vi "pf_Get_3D-Data_3D03.vi"(7 "Aquired Image":T1, 8 "error in (no error)":errorcluster, 9 "FrameCombine_NrOfFrames":u32, 10 "FrameCombine_Enable":bool=TRUE, 11 "PeakDetector_Mode":u32) -> (0 "error out":errorcluster, 1 "Quality Profile":u8[][](array[numeric]), 2 "Width Profile":u8[][](array[numeric]), 3 "Peak Profile":sgl[][](array[numeric]), 4 "Linescan":u8[][](array[numeric]), 5 "Status Line":u8[][](array[numeric]))   [LabVIEW 2012, in "Photonfocus_Toolkit.lvlib"]
uses:
  <userlib>/Photonfocus Toolkit/Photonfocus_Toolkit.lvlib
  <vilib>/vision/Image Controls.llb/IMAQ Image.ctl
  <vilib>/Analysis/Matrix/Numeric/Conversions/Array To Matrix - RA2.vi
  <vilib>/Analysis/Matrix/Numeric/Conversions/Matrix To Array - RM.vi
  <vilib>/Analysis/Matrix/NI_Matrix.lvlib
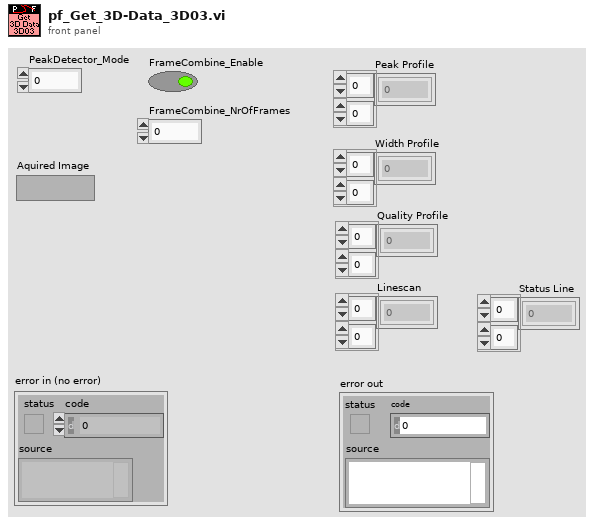
[diagram p1: front panel]
types:
  T1 = typedef "IMAQ Image.ctl" = refnum<image>
  T2 = enum8{"2D only", "2D and 3D", "3D only", "Undefined"}
  T3 = typedef "NI_Matrix.lvlib/RealMatrix.ctl" = dbl[][]
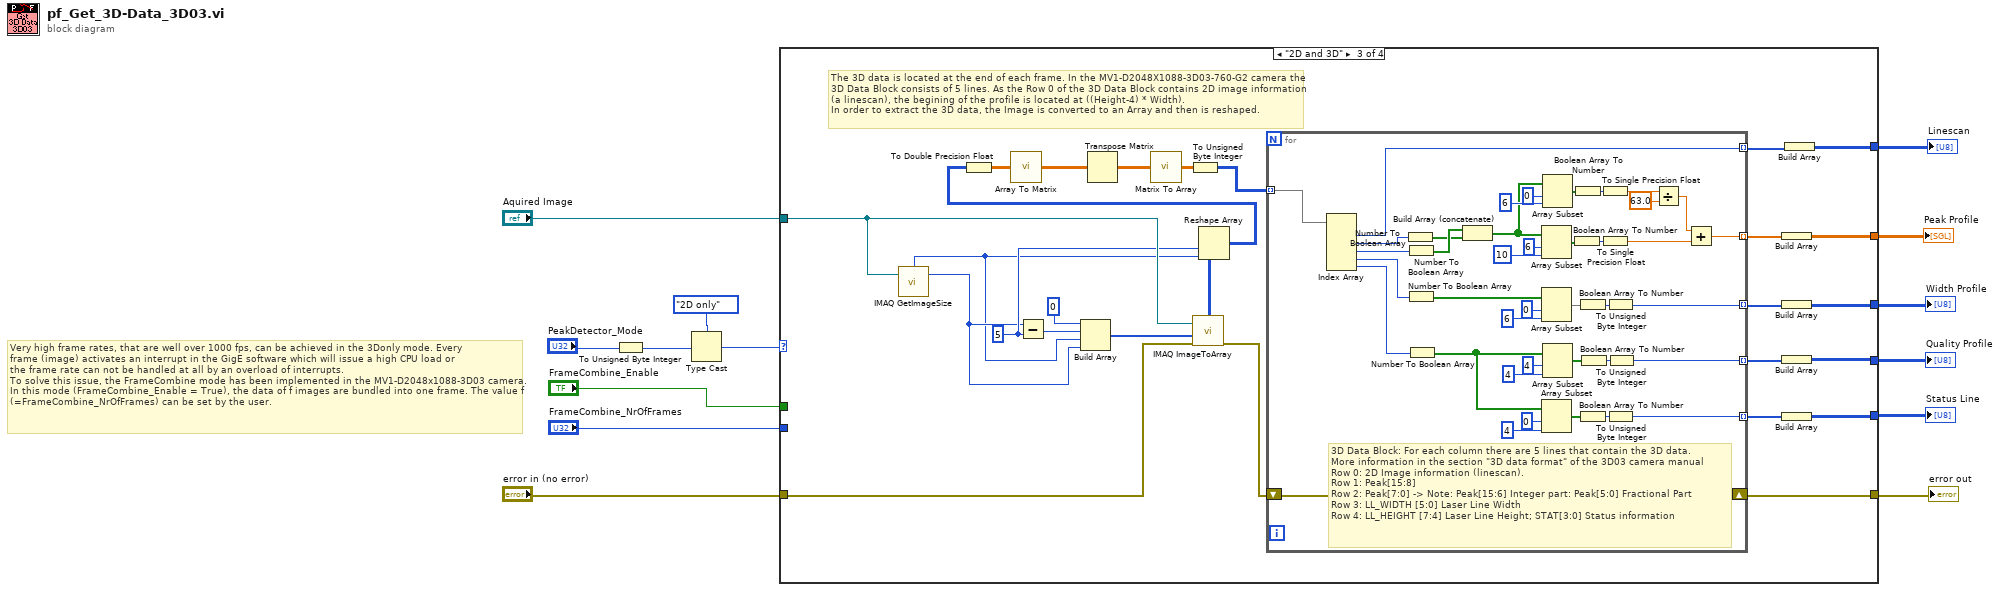
[diagram p0: block diagram]
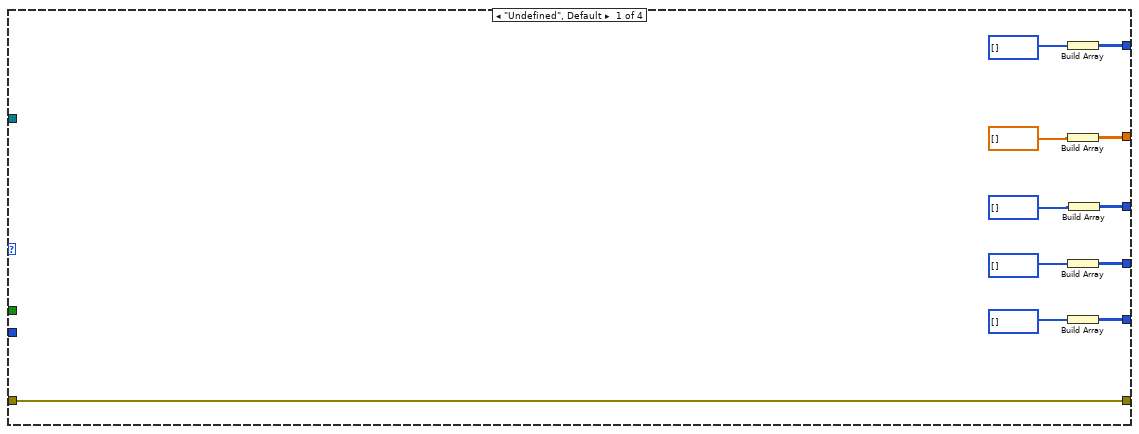
[diagram p2: hidden frame]
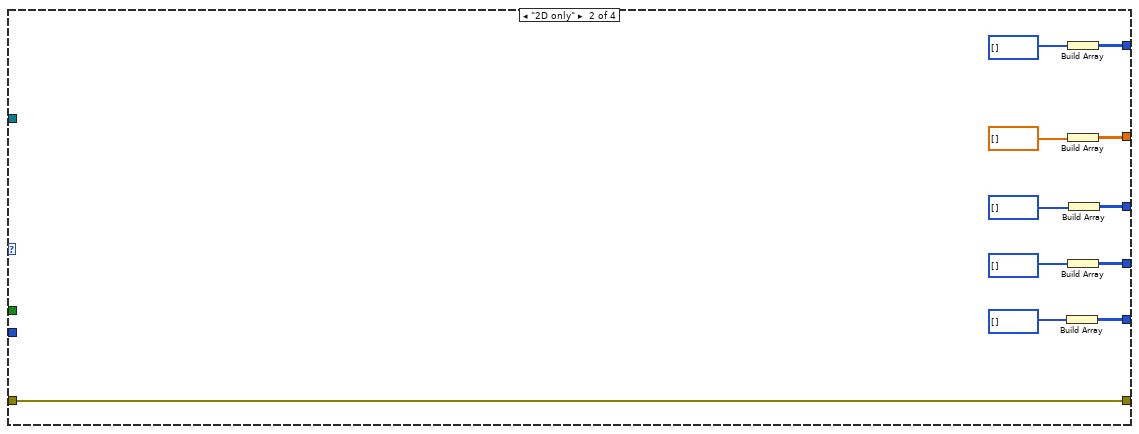
[diagram p3: hidden frame]
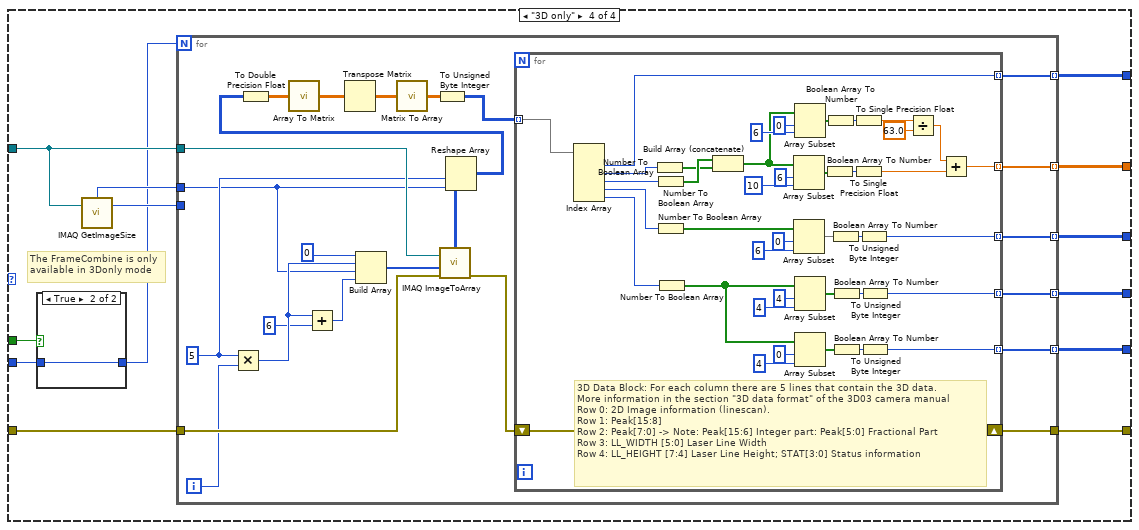
[diagram p4: hidden frame]
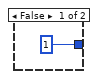
[diagram p5: hidden frame]
diagram:
  # "Very high frame rates, that are well over 1000 fps, can be achieved in the 3Donly mode. Every\nframe (image) activates an interrupt in the GigE software which will issue a high CPU load or\nthe frame rate can not be handled at all by an overload of interrupts.\nTo solve this issue, the FrameCombine mode has been implemented in the MV1-D2048x1088-3D03 camera. In this mode (FrameCombine_Enable = True), the data of f images are bundled into one frame. The value f (=FrameCombine_NrOfFrames) can be set by the user."
  n1 = To Unsigned Byte Integer(number="PeakDetector_Mode") -> (unsigned 8bit integer=w7:u8)
  n2 = Type Cast(type=T2."2D only", x=w7) -> (*(type *) &x=w9:T2)
  n3 = case shown="\"2D and 3D\"" w9 {
    tunnel: "Aquired Image" -> [_ _ w56 w116]
    tunnel: [w21 w34 w47 w112] -> w5
    tunnel: [w20 w32 w45 w111] -> w4
    tunnel: [w19 w31 w43 w110] -> w3
    tunnel: [w25 w36 w62 w109] -> w13
    tunnel: "FrameCombine_NrOfFrames" -> [_ _ _ w107]
    tunnel: "error in (no error)" -> [w25 w36 w57 w113]
    tunnel: "FrameCombine_Enable" -> [_ _ _ w108]
    tunnel: [w17 w28 w41 w105] -> w2
    tunnel: [w15 w26 w37 w104] -> w1
    frame "Undefined", Default {
      n4 = Build Array(u8[] []) -> (w17:u8[][])
      n5 = Build Array(sgl[] []) -> (w21:sgl[][])
      n6 = Build Array(u8[] []) -> (w19:u8[][])
      n7 = Build Array(u8[] []) -> (w15:u8[][])
      n8 = Build Array(u8[] []) -> (w20:u8[][])
    }
    frame "2D only" {
      n9 = Build Array(u8[] []) -> (w26:u8[][])
      n10 = Build Array(u8[] []) -> (w28:u8[][])
      n11 = Build Array(sgl[] []) -> (w34:sgl[][])
      n12 = Build Array(u8[] []) -> (w31:u8[][])
      n13 = Build Array(u8[] []) -> (w32:u8[][])
    }
    frame "2D and 3D" {
      w55 = 5 ("y")
      # "The 3D data is located at the end of each frame. In the MV1-D2048X1088-3D03-760-G2 camera the 3D Data Block consists of 5 lines. As the Row 0 of the 3D Data Block contains 2D image information (a linescan), the begining of the profile is located at ((Height-4) * Width).\nIn order to extract the 3D data, the Image is converted to an Array and then is reshaped."
      n14 = call "IMAQ GetImageSize"("Image"=w56) -> ("Y Resolution"=w40:i32, "X Resolution"=w39:i32)  [unwired: 3 in, 1 out]
      n15 = Subtract(x=w40, y=w55) -> (x-y=w60:i32)
      n16 = Build Array "Build Array"(0, w60, w39, w40) -> (w58:i32[])
      n17 = call "IMAQ ImageToArray"("error in (no error)"=w57, "Optional Rectangle"=w58, "Image"=w56) -> ("error out"=w63:errorcluster, "Image Pixels (U8)"=w59:u8[][])  [unwired: 4 out]
      n18 = Reshape Array "Reshape Array"(w59, w55, w39) -> (w52:u8[][])
      n19 = To Double Precision Float(number=w52) -> (double precision float=w51:dbl[][])
      n20 = call-poly <vilib>:"Array To Matrix.vi"("Real 2D Array"=w51) -> ("Real Matrix"=w54:T3)
      n21 = Transpose Matrix(1:w54) -> (0:w53:T3)
      n22 = call-poly <vilib>:"Matrix To Array.vi"("Real Matrix"=w53) -> ("Real 2D Array"=w49:dbl[][])
      n23 = To Unsigned Byte Integer(number=w49) -> (unsigned 8bit integer=w50:u8[][])
      n24 = for {
        shift-right: [w82] -> w62
        shift-left: w63 -> [w82]
        tunnel: [w83] -> w48 mode=indexing
        tunnel: w50 -> [w81] mode=indexing
        tunnel: [w80] -> w46 mode=indexing
        tunnel: [w75] -> w44 mode=indexing
        tunnel: [w70] -> w42 mode=indexing
        tunnel: [w64] -> w38 mode=indexing
        # "3D Data Block: For each column there are 5 lines that contain the 3D data.\nMore information in the section \"3D data format\" of the 3D03 camera manual\nRow 0: 2D Image information (linescan).\nRow 1: Peak[15:8]\nRow 2: Peak[7:0] -> Note: Peak[15:6] Integer part: Peak[5:0] Fractional Part\nRow 3: LL_WIDTH [5:0] Laser Line Width\nRow 4: LL_HEIGHT [7:4] Laser Line Height; STAT[3:0] Status information"
        n25 = Index Array "Index Array"(array=w81) -> (element #1=w70:u8, element #2=w71:u8, element #3=w72:u8, element #4=w73:u8, element #5=w74:u8)  [unwired: 5 in]
        n26 = Number To Boolean Array(number=w71) -> (Boolean array=w91:bool[])
        n27 = Number To Boolean Array(number=w72) -> (Boolean array=w92:bool[])
        n28 = Number To Boolean Array(number=w73) -> (Boolean array=w84:bool[])
        n29 = Number To Boolean Array(number=w74) -> (Boolean array=w65:bool[])
        n30 = Build Array (concatenate) "Build Array"(w92, w91) -> (w93:bool[])
        n31 = Array Subset(array=w93, index=6, length=10) -> (w98:bool[])
        n32 = Array Subset(array=w84, index=0, length=6) -> (w85:bool[])
        n33 = Array Subset(array=w65, index=0, length=4) -> (w67:bool[])
        n34 = Array Subset "Array Subset"(array=w93, index=0, length=6) -> (w99:bool[])
        n35 = Array Subset(array=w65, index=4, length=4) -> (w77:bool[])
        n36 = Boolean Array To Number(Boolean array=w98) -> (number=w94:u32)
        n37 = Boolean Array To Number(Boolean array=w99) -> (number=w96:u32)
        n38 = Boolean Array To Number(Boolean array=w85) -> (number=w86:u32)
        n39 = Boolean Array To Number(Boolean array=w67) -> (number=w66:u32)
        n40 = Boolean Array To Number(Boolean array=w77) -> (number=w76:u32)
        n41 = To Single Precision Float(number=w96) -> (single precision float=w90:sgl)
        n42 = To Single Precision Float(number=w94) -> (single precision float=w89:sgl)
        n43 = To Unsigned Byte Integer(number=w86) -> (unsigned 8bit integer=w80:u8)
        n44 = To Unsigned Byte Integer(number=w66) -> (unsigned 8bit integer=w64:u8)
        n45 = To Unsigned Byte Integer(number=w76) -> (unsigned 8bit integer=w75:u8)
        n46 = Divide(x=w90, y=sgl 63.0) -> (x/y=w95:sgl)
        n47 = Add(x=w95, y=w89) -> (x+y=w83:sgl)
      }
      n48 = Build Array(w48) -> (w47:sgl[][])
      n49 = Build Array(w46) -> (w45:u8[][])
      n50 = Build Array(w44) -> (w43:u8[][])
      n51 = Build Array(w38) -> (w37:u8[][])
      n52 = Build Array(w42) -> (w41:u8[][])
    }
    frame "3D only" {
      # "The FrameCombine is only available in 3Donly mode"
      n53 = case shown="True" w108 {
        tunnel: w107 -> [_ w118]
        tunnel: [1 w118] -> w106
        frame False {
        }
        frame True {
        }
      }
      n54 = call "IMAQ GetImageSize"("Image"=w116) -> ("Y Resolution"=w114:i32, "X Resolution"=w115:i32)  [unwired: 3 in, 1 out]
      n55 = for {
        N: w106 -> [_]
        tunnel: w116 -> [w132]
        tunnel: w115 -> [w121]
        tunnel: w114 -> [_]
        tunnel: w113 -> [w131]
        tunnel: [w127] -> w109
        tunnel: [w130] -> w112 mode=indexing
        tunnel: [w129] -> w111 mode=indexing
        tunnel: [w128] -> w110 mode=indexing
        tunnel: [w123] -> w105 mode=indexing
        tunnel: [w119] -> w104 mode=indexing
        i -> [w126]
        w122 = 5 ("y")
        n56 = Multiply(x=w122, y=w126) -> (x*y=w124:i32)
        n57 = Add(x=w124, y=6) -> (x+y=w125:i32)
        n58 = Build Array "Build Array"(0, w124, w121, w125) -> (w139:i32[])
        n59 = call "IMAQ ImageToArray"("error in (no error)"=w131, "Optional Rectangle"=w139, "Image"=w132) -> ("error out"=w142:errorcluster, "Image Pixels (U8)"=w140:u8[][])  [unwired: 4 out]
        n60 = Reshape Array "Reshape Array"(w140, w122, w121) -> (w136:u8[][])
        n61 = To Double Precision Float(number=w136) -> (double precision float=w135:dbl[][])
        n62 = call-poly <vilib>:"Array To Matrix.vi"("Real 2D Array"=w135) -> ("Real Matrix"=w138:T3)
        n63 = Transpose Matrix(1:w138) -> (0:w137:T3)
        n64 = call-poly <vilib>:"Matrix To Array.vi"("Real Matrix"=w137) -> ("Real 2D Array"=w133:dbl[][])
        n65 = To Unsigned Byte Integer(number=w133) -> (unsigned 8bit integer=w134:u8[][])
        n66 = for {
          shift-right: [w161] -> w127
          shift-left: w142 -> [w161]
          tunnel: [w162] -> w130 mode=indexing
          tunnel: w134 -> [w160] mode=indexing
          tunnel: [w159] -> w129 mode=indexing
          tunnel: [w154] -> w128 mode=indexing
          tunnel: [w149] -> w123 mode=indexing
          tunnel: [w143] -> w119 mode=indexing
          # "3D Data Block: For each column there are 5 lines that contain the 3D data.\nMore information in the section \"3D data format\" of the 3D03 camera manual\nRow 0: 2D Image information (linescan).\nRow 1: Peak[15:8]\nRow 2: Peak[7:0] -> Note: Peak[15:6] Integer part: Peak[5:0] Fractional Part\nRow 3: LL_WIDTH [5:0] Laser Line Width\nRow 4: LL_HEIGHT [7:4] Laser Line Height; STAT[3:0] Status information"
          n67 = Index Array "Index Array"(array=w160) -> (element #1=w149:u8, element #2=w150:u8, element #3=w151:u8, element #4=w152:u8, element #5=w153:u8)  [unwired: 5 in]
          n68 = Number To Boolean Array(number=w150) -> (Boolean array=w170:bool[])
          n69 = Number To Boolean Array(number=w151) -> (Boolean array=w171:bool[])
          n70 = Number To Boolean Array(number=w152) -> (Boolean array=w163:bool[])
          n71 = Number To Boolean Array(number=w153) -> (Boolean array=w144:bool[])
          n72 = Build Array (concatenate) "Build Array"(w171, w170) -> (w172:bool[])
          n73 = Array Subset(array=w172, index=6, length=10) -> (w177:bool[])
          n74 = Array Subset(array=w163, index=0, length=6) -> (w164:bool[])
          n75 = Array Subset "Array Subset"(array=w172, index=0, length=6) -> (w178:bool[])
          n76 = Array Subset(array=w144, index=4, length=4) -> (w156:bool[])
          n77 = Array Subset(array=w144, index=0, length=4) -> (w146:bool[])
          n78 = Boolean Array To Number(Boolean array=w177) -> (number=w173:u32)
          n79 = Boolean Array To Number(Boolean array=w178) -> (number=w175:u32)
          n80 = Boolean Array To Number(Boolean array=w164) -> (number=w165:u32)
          n81 = Boolean Array To Number(Boolean array=w156) -> (number=w155:u32)
          n82 = Boolean Array To Number(Boolean array=w146) -> (number=w145:u32)
          n83 = To Single Precision Float(number=w175) -> (single precision float=w169:sgl)
          n84 = To Single Precision Float(number=w173) -> (single precision float=w168:sgl)
          n85 = To Unsigned Byte Integer(number=w165) -> (unsigned 8bit integer=w159:u8)
          n86 = To Unsigned Byte Integer(number=w155) -> (unsigned 8bit integer=w154:u8)
          n87 = To Unsigned Byte Integer(number=w145) -> (unsigned 8bit integer=w143:u8)
          n88 = Divide(x=w169, y=sgl 63.0) -> (x/y=w174:sgl)
          n89 = Add(x=w174, y=w168) -> (x+y=w162:sgl)
        }
      }
    }
  }
  "error out" <- w13
  "Peak Profile" <- w5
  "Width Profile" <- w4
  "Quality Profile" <- w3
  "Linescan" <- w2
  "Status Line" <- w1
